vi "oa_Check Data for Waveform Reference (1 Channel).vi"(0 "resampled signal":cluster{"r0":dbl, "dr":dbl, "Y":dbl[]}={"r0"=0.0, "dr"=1.0, "Y"=[]} {"r0" format="%.2p"; "dr" format="%.2p"; "Y" format="%.2f"}, 1 "reset? (True)":bool=TRUE, 5 "select reference data":T2(ring), 7 "speed profile":T1 {"speed [RPM]" format="%.2f"; "time [s]" format="%.2f"}, 9 "interpolated pulse positions":dbl[](array[numeric]) format="%.2f", 11 "error in (no error)":errorcluster, 12 "even angle reference in":cluster{"r0":dbl, "dr":dbl, "Y":dbl[]}={"r0"=0.0, "dr"=1.0, "Y"=[]} {"r0" format="%.2p"; "dr" format="%.2p"; "Y" format="%.2f"}) -> (2 "empty signal?":bool, 3 "reset":bool, 4 "resampled signal out":cluster{"r0":dbl, "dr":dbl, "Y":dbl[]}={"r0"=0.0, "dr"=1.0, "Y"=[]} {"r0" format="%.2p"; "dr" format="%.2p"; "Y" format="%.2f"}, 6 "select reference dataout":T2(ring), 8 "speed profile out":T1 {"speed [RPM]" format="%.2f"; "time [s]" format="%.2f"}, 10 "interpolated pulse positions out":dbl[](array[numeric]) format="%.2f", 14 "even angle reference out":cluster{"r0":dbl, "dr":dbl, "Y":dbl[]}={"r0"=0.0, "dr"=1.0, "Y"=[]} {"r0" format="%.2p"; "dr" format="%.2p"; "Y" format="%.2f"}, 15 "error out":errorcluster)   [LabVIEW 2017, in "SoundVib_Resampling.lvlib"]
uses:
  <vilib>/addons/Sound and Vibration/Order Analysis/Resample Order Tracking/SoundVib_Resampling.lvlib
  <vilib>/addons/Sound and Vibration/Order Analysis/Tach Process/SubVIs/speed profile.ctl
  <vilib>/addons/Sound and Vibration/Order Analysis/Resample Order Tracking/SubVIs/OAT Verify Resampled Signal (Single Channel).vi
  <vilib>/addons/Sound and Vibration/Order Analysis/Tach Process/SoundVib_TachProcess.lvlib
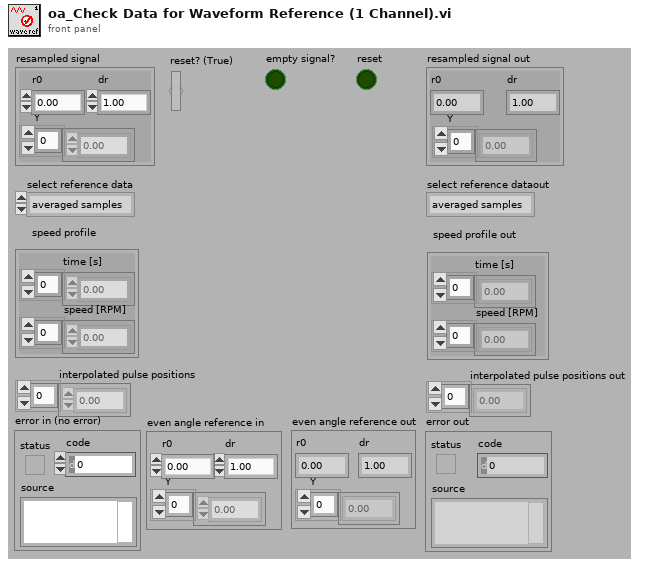
[diagram p1: front panel]
types:
  T1 = typedef "SoundVib_TachProcess.lvlib/speed profile.ctl" = cluster{"time [s]":dbl[], "speed [RPM]":dbl[]}
  T2 = enum16{"averaged samples", "initial samples", "final samples"}
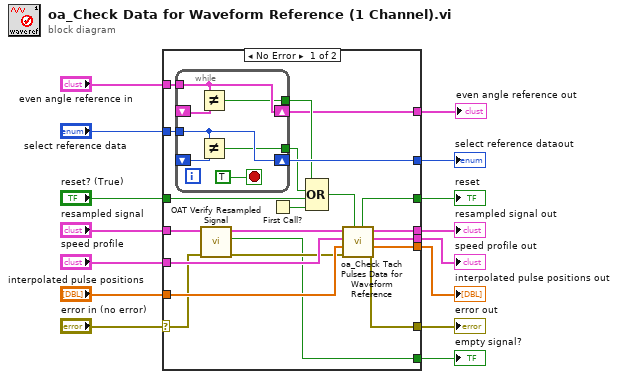
[diagram p0: block diagram]
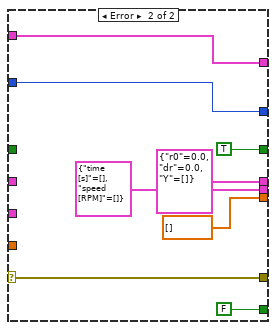
[diagram p2: hidden frame]
diagram:
  n1 = case shown="No Error" "error in (no error)" {
    selector: "error in (no error)" -> [w23 w51]
    tunnel: [w26 w51] -> w14
    tunnel: "select reference data" -> [w36 w50]
    tunnel: "reset? (True)" -> [w34 _]
    tunnel: [w35 w50] -> w11
    tunnel: "resampled signal" -> [w17 _]
    tunnel: "speed profile" -> [w31 _]
    tunnel: "interpolated pulse positions" -> [w30 _]
    tunnel: [w29 cluster{"r0":dbl, "dr":dbl, "Y":dbl[]} {"r0"=0.0, "dr"=0.0, "Y"=[]} ("resampled signal out")] -> w7
    tunnel: [w28 T1 {"time [s]"=[], "speed [RPM]"=[]} ("speed profile out")] -> w6
    tunnel: [w27 dbl[] [] ("interpolated pulse positions out")] -> w5
    tunnel: [w25 TRUE ("reset")] -> w4
    tunnel: "even angle reference in" -> [w21 w45]
    tunnel: [w19 w45] -> w2
    tunnel: [w18 FALSE ("empty signal?")] -> w1
    frame No Error {
      n2 = while {
        shift-right: [w43] -> w35
        shift-left: _ -> [w42]
        tunnel: w36 -> [w43]
        tunnel: [w40] -> w33
        tunnel: w21 -> [w38]
        shift-right: [w38] -> w19
        shift-left: _ -> [w39]
        tunnel: [w37] -> w20
        stop <- TRUE stop-if-true
        n3 = Not Equal?(x=w38, y=w39) -> (x != y?=w37:bool)
        n4 = Not Equal?(x=w43, y=w42) -> (x != y?=w40:bool)
      }
      n5 = call-poly <vilib>:"OAT Verify Resampled Signal.vi"("error in (no error)"=w23, "resampled signal"=w17) -> ("error out"=w22:errorcluster, "empty signal?"=w18:bool, "resampled signal dup"=w16:cluster{"r0":dbl, "dr":dbl, "Y":dbl[]})  [unwired: 7 in]
      n6 = First Call?() -> (First Call?: T/F=w24:bool)
      n7 = Compound Arithmetic op=OR(w20, w33, w34, w24) -> (w32:bool)
      n8 = call <vilib>:"oa_Check Tach Pulses Data for Waveform Reference.vi"("reset? (True)"=w32, "error in (no error)"=w22, "interpolated pulse positions"=w30, "speed profile"=w31, "resampled signal"=w16) -> ("error out"=w26:errorcluster, "interpolated pulse positions out"=w27:dbl[], "speed profile out"=w28:T1, "resampled signal out"=w29:cluster{"r0":dbl, "dr":dbl, "Y":dbl[]}, "reset"=w25:bool)  [unwired: 2 in]
    }
    frame Error {
    }
  }
  "select reference dataout" <- w11
  "interpolated pulse positions out" <- w5
  "speed profile out" <- w6
  "error out" <- w14
  "reset" <- w4
  "resampled signal out" <- w7
  "even angle reference out" <- w2
  "empty signal?" <- w1
